vi "Measure Sound from Digital Mic - PDM.vi"() -> ()   [LabVIEW 2022 SP3]
doc: "This example performs a continuous acquisition of PCM data. At the same time, the GPIO lines are used for digital input and digital output."
uses:
  <vilib>/PDM Acquisition Toolkit/host/Classes/Session/Controls/Logic Levels.ctl
  <vilib>/PDM Acquisition Toolkit/shared/controls/decimation order.ctl
  <vilib>/PDM Acquisition Toolkit/host/Classes/Tasks/PDM Tasks/Controls/Acquisition Mode.ctl
  <vilib>/PDM Acquisition Toolkit/shared/controls/clock mode.ctl
  <vilib>/addons/_NISVFA/_Shared subVIs/Common/SVL Set dB Reference (1 Ch).vi
  <vilib>/addons/Sound and Vibration/svt_Level/SVL AC & DC Level (Time) (1 Ch).vi
  <vilib>/addons/_NISVFA/_Shared subVIs/Common/SVL Set dB Reference (variant).vi
  <vilib>/addons/_NISVFA/_Shared subVIs/Common/svc_Get SV Channel Info.vi
  <vilib>/Analysis/baseanly.llb/Mean.vi
  <vilib>/Analysis/baseanly.llb/Mean (DBL).vi
  <vilib>/addons/_NISVFA/_Shared subVIs/Windowing/svfa_Scaled Time Domain Window (Array).vi
  <vilib>/addons/_NISVFA/_Shared subVIs/Common/svc_Unit Label to Engineering Units.vi
  <vilib>/addons/_NISVFA/_Shared subVIs/Common/svc_Engineering Units to Unit Label.vi
  <vilib>/addons/_NISVFA/_Spectrum Processing/subVIs/svfa_Spectrum Info Window to windowTd Type Def.vi
  <vilib>/Analysis/4window.llb/Force Window.vi
  <vilib>/Analysis/4window.llb/Force Window (DBL).vi
  <vilib>/Analysis/4window.llb/Exponential Window.vi
  <vilib>/Analysis/4window.llb/Exponential Window (DBL).vi
  <vilib>/PDM Acquisition Toolkit/host/API/Public/Create Tasks/Create PDM Input Task.vi
  <vilib>/PDM Acquisition Toolkit/host/API/Public/Configure/Timing/Configure Timing - PDM Input.vi
  <vilib>/PDM Acquisition Toolkit/host/API/Public/Configure/PDM Channel/Configure Microphone Sensitivity DBFS.vi
  <vilib>/PDM Acquisition Toolkit/host/API/Public/Read/Read PCM Waveform.vi
  <vilib>/addons/_NISVFA/_Shared subVIs/Common/svc_Caller VI Returned in Error Source.vi
  <vilib>/addons/_NISVFA/_Shared subVIs/Common/svc_Get Window Info.vi
  <vilib>/Analysis/0measdsp.llb/Scaled Time Domain Window.vi
  <vilib>/Analysis/0measdsp.llb/Scaled Time Domain Window (DBL).vi
  <vilib>/Utility/error.llb/Error Cluster From Error Code.vi
  <vilib>/Analysis/baseanly.llb/Std Deviation and Variance.vi
  <vilib>/addons/Sound and Vibration/svt_Weighting/SVT Weighting Filter (1 Ch).vi
  <vilib>/addons/Sound and Vibration/svt_Level/SVL Leq Sound Level (1 Ch).vi
  <vilib>/PDM Acquisition Toolkit/host/API/Public/Clear/Clear PDM Input Task.vi
  <vilib>/PDM Acquisition Toolkit/host/API/PDM Acquisition Toolkit.lvlib
  <vilib>/PDM Acquisition Toolkit/host/Classes/Tasks/PDM Tasks/PDM Task.lvclass
  <vilib>/PDM Acquisition Toolkit/shared/PDM Shared.lvlib
  <vilib>/addons/Sound and Vibration/svt_Weighting/SoundVib_ABCWeighting.lvlib
  <vilib>/addons/Sound and Vibration/svt_Level/SoundVib_SoundLevel.lvlib
  <vilib>/PDM Acquisition Toolkit/host/Classes/Session/DecoderSession.lvclass
panel:
  out "Leq sound level [dB EU]":dbl=63.21387111345029 format="%.2f"
  in  "weighting":u16(ring) items=["Linear", "A-weighting", "B-weighting", "C-weighting"]
  out "Error Out":errorcluster
  out "Actual PCM Clock Rate":dbl=47999.99987881165 format="%#_6p"
  out "Actual PDM Clock Rate":dbl=3071999.9922439456 format="%#_6p"
  out "Waveform Graph":waveform(dbl)(graph)={"t0"=timestamp(0 s since 1904-01-01), "dt"=2.0833333385932442e-05, "Y"=[], "attributes"=variant("NI_ChannelName"=variant(string "PDMI0L"), "NI_dBReference"=variant(dbl 2e-05))}
  in  "Number of Samples":i32=12000
  in  "PDM Clock Rate":dbl=3072000.0 format="%#_6p"
  in  "PDM Channels":string="PXI1Slot5\\PDMi 0"
  in  "Logic Level":T1
  in  "Decimation Factor":T2=64 items=["24"=24, "32"=32, "48"=48, "64"=64, "96"=96, "128"=128]
  in  "Microphone Sensitivity (dBFS)":dbl=-26.0 format="%#_13g"
  in  "Stop":bool
  # "PDM Input"
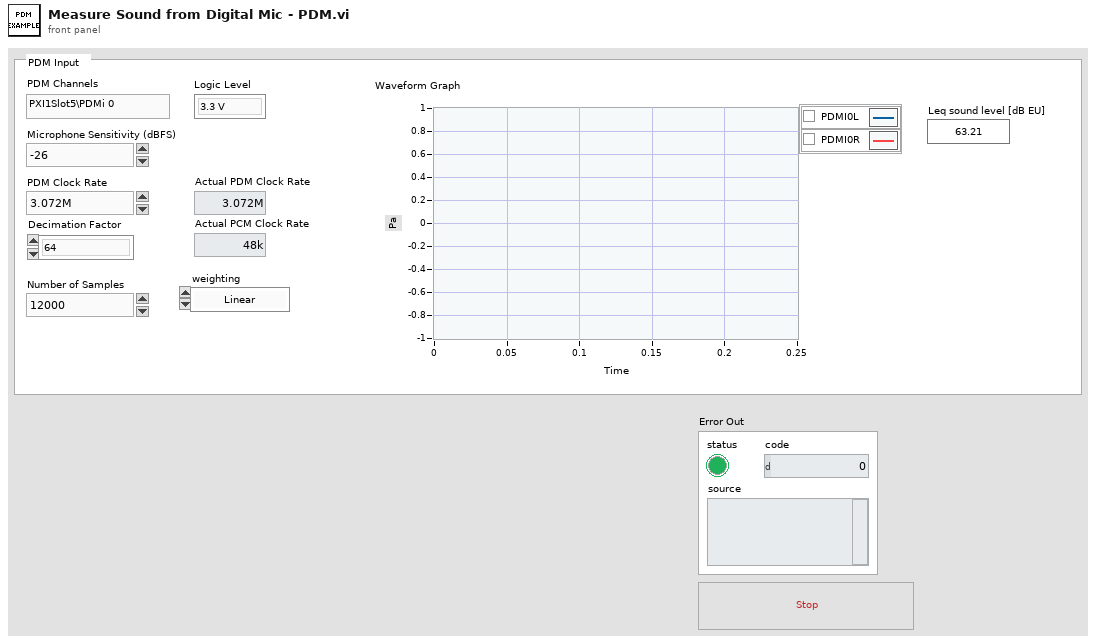
[diagram p1: front panel]
types:
  T1 = typedef "PDM Acquisition Class Library.lvlib/DecoderSession.lvclass/Logic Levels.ctl" = enum16{"3.3 V", "1.8 V", "1.2 V"}
  T2 = typedef "PDM Shared.lvlib/decimation order.ctl" = u16
  T3 = typedef "PDM Shared.lvlib/clock mode.ctl" = enum16{"divided clock", "DDS"}
  T4 = typedef "PDM Acquisition Class Library.lvlib/PDM Task.lvclass/Acquisition Mode.ctl" = enum16{"Finite", "Continuous"}
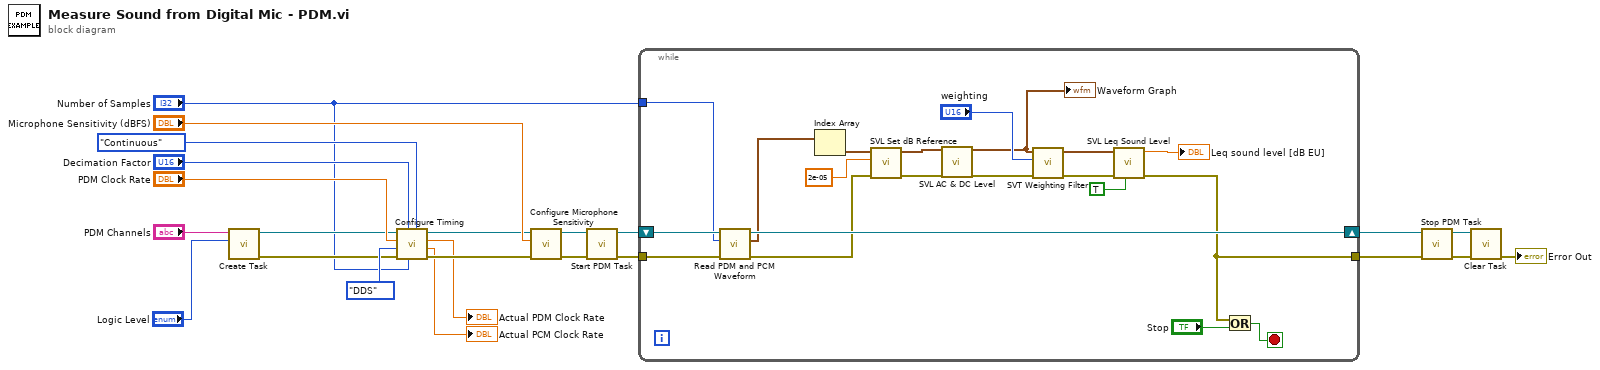
[diagram p0: block diagram]
diagram:
  n1 = call-poly <vilib>:"Create Task.vi"("logic level"="Logic Level", "channel list"="PDM Channels") -> ("error out"=w6:errorcluster, "PDM input task out"=w7:refnum<data-value>)  [unwired: 8 in]
  n2 = call-poly <vilib>:"Configure Timing.vi"("acquisition mode"=Acquisition_Mode."Continuous" ("Acquisition Mode"), "number of PCM samples"="Number of Samples", "decimation factor"="Decimation Factor", "error in"=w6, "clock mode"=clock_mode."DDS" ("Clock Type"), "PDM clock rate"="PDM Clock Rate", "PDM input task in"=w7) -> ("error out"=w12:errorcluster, "actual PCM clock rate"=→"Actual PCM Clock Rate":dbl, "actual PDM clock rate"=→"Actual PDM Clock Rate":dbl, "PDM input task out"=w13:refnum<data-value>)  [unwired: 1 in]
  n3 = call-poly <vilib>:"Configure Microphone Sensitivity.vi"("error in"=w12, "microphone sensitivity (dBFS)"="Microphone Sensitivity (dBFS)", "PDM input task in"=w13) -> ("error out"=w10:errorcluster, "PDM input task out"=w11:refnum<data-value>)  [unwired: 7 in]
  n4 = call <vilib>:"Start PDM Task.vi"("error in"=w10, "PDM input task in"=w11) -> ("error out"=w18:errorcluster, "PDM input task out"=w19:refnum<data-value>)  [unwired: 8 in]
  n5 = while {
    tunnel: w18 -> [w41]
    tunnel: "Number of Samples" -> [w40]
    shift-right: [w43] -> w22
    shift-left: w19 -> [w42]
    tunnel: [w24] -> w1
    stop <- w39 stop-if-true
    n6 = call-poly <vilib>:"Read PDM and PCM Waveform.vi"("error in"=w41, "samples per channel"=w40, "PDM input task in"=w42) -> ("error out"=w31:errorcluster, "PCM waveforms"=w29:waveform(dbl)[], "PDM input task out"=w43:refnum<data-value>)  [unwired: 5 in, 1 out]
    n7 = Index Array(array=w29) -> (element=w32:waveform(dbl))  [unwired: 1 in]
    n8 = call-poly <vilib>:"SVL Set dB Reference.vi"("error in (no error)"=w31, "dB reference [EU]"=2e-05, "scaled signal in [EU]"=w32) -> ("error out"=w25:errorcluster, "scaled signal out [EU]"=w28:waveform(dbl))  [unwired: 7 in]
    n9 = call-poly <vilib>:"SVL AC & DC Level.vi"("scaled signal [EU]"=w28, "error in (no error)"=w25) -> ("AC signal [EU]"=w27:waveform(dbl), "error out"=w26:errorcluster)  [unwired: 12 in, 4 out]
    "Waveform Graph" <- w27
    n10 = call-poly <vilib>:"SVT Weighting Filter.vi"("error in (no error)"=w26, "weighting"="weighting", "scaled signal [EU]"=w27) -> ("error out"=w36:errorcluster, "weighted signal [EU]"=w33:waveform(dbl))  [unwired: 6 in]
    n11 = call-poly <vilib>:"SVL Leq Sound Level.vi"("restart averaging (F)"=TRUE, "error in (no error)"=w36, "scaled signal [EU]"=w33) -> ("error out"=w24:errorcluster, "Leq sound level [dB EU]"=→"Leq sound level [dB EU]":dbl)  [unwired: 6 in, 1 out]
    n12 = Or(x=w24, y="Stop") -> (x .or. y?=w39:bool)
  }
  n13 = call <vilib>:"Stop PDM Task.vi"("error in"=w1, "PDM input task in"=w22) -> ("error out"=w9:errorcluster, "PDM input task out"=w21:refnum<data-value>)  [unwired: 8 in]
  n14 = call-poly <vilib>:"Clear Task.vi"("error in"=w9, "PDM input task in"=w21) -> ("error out"=→"Error Out":errorcluster)  [unwired: 9 in]
